vi "VBus Set from X Y Rot Angle Inputs_Cartesian.vi"(6 "Rotation":dbl, 7 "Gyro Angle":dbl, 8 "Error":errorcluster, 9 "Y":dbl, 10 "X":dbl, 11 "RobotDriveDevRef":T1={"DevStatus"={"status"=FALSE, "code"=0, "source"=""}, "Motors[]"=[], "Square Inputs"=FALSE, "Max Output"=1.0}) -> (0 "Error Out":errorcluster, 3 "RobotDriveDevRef Out":T1={"DevStatus"={"status"=FALSE, "code"=0, "source"=""}, "Motors[]"=[], "Square Inputs"=FALSE, "Max Output"=1.0})   [LabVIEW 2017, in "MechamunDrive.lvlib"]
doc: "Configures the motors for holonomic driving. Holonomic driving allows you to move the robot in any direction without first rotating or maneuvering the robot.\n\nThis VI requires the robot to have either four omni-directional wheels and four motors mounted at 45 degree angles in the four corners of a square frame or to have four mecanum wheels driven by four motors.\n\nThe control input is intended to be connected directly to the X, Y, and Z axes of a joystick. The Y axis is inverted for you.\n\nThis software is licensed. Open the labview\\readme\\WPI Robotics Library Open Source License.txt file for more information."
uses:
  MechamunDrive.lvlib
  <vilib>/Rock Robotics/WPI/RobotDrive/WPI_RobotDriveDevRef.ctl
  <vilib>/Rock Robotics/WPI/MotorControl/WPI_MotorControlDeviceRef.ctl
  <vilib>/Rock Robotics/WPI/MotorControl/WPI_MotorControlType.ctl
  <vilib>/Rock Robotics/SystemInterfaces/DIO/FPGA_DIOPWMChannel.ctl
  <vilib>/Rock Robotics/WPI/PWM/WPI_PWMDeadband.ctl
  <vilib>/Rock Robotics/SystemInterfaces/DIO/FPGA_DIOChannel.ctl
  <vilib>/Rock Robotics/SystemInterfaces/NetworkCommunication/NetComm_UsageReport_ResourceType.ctl
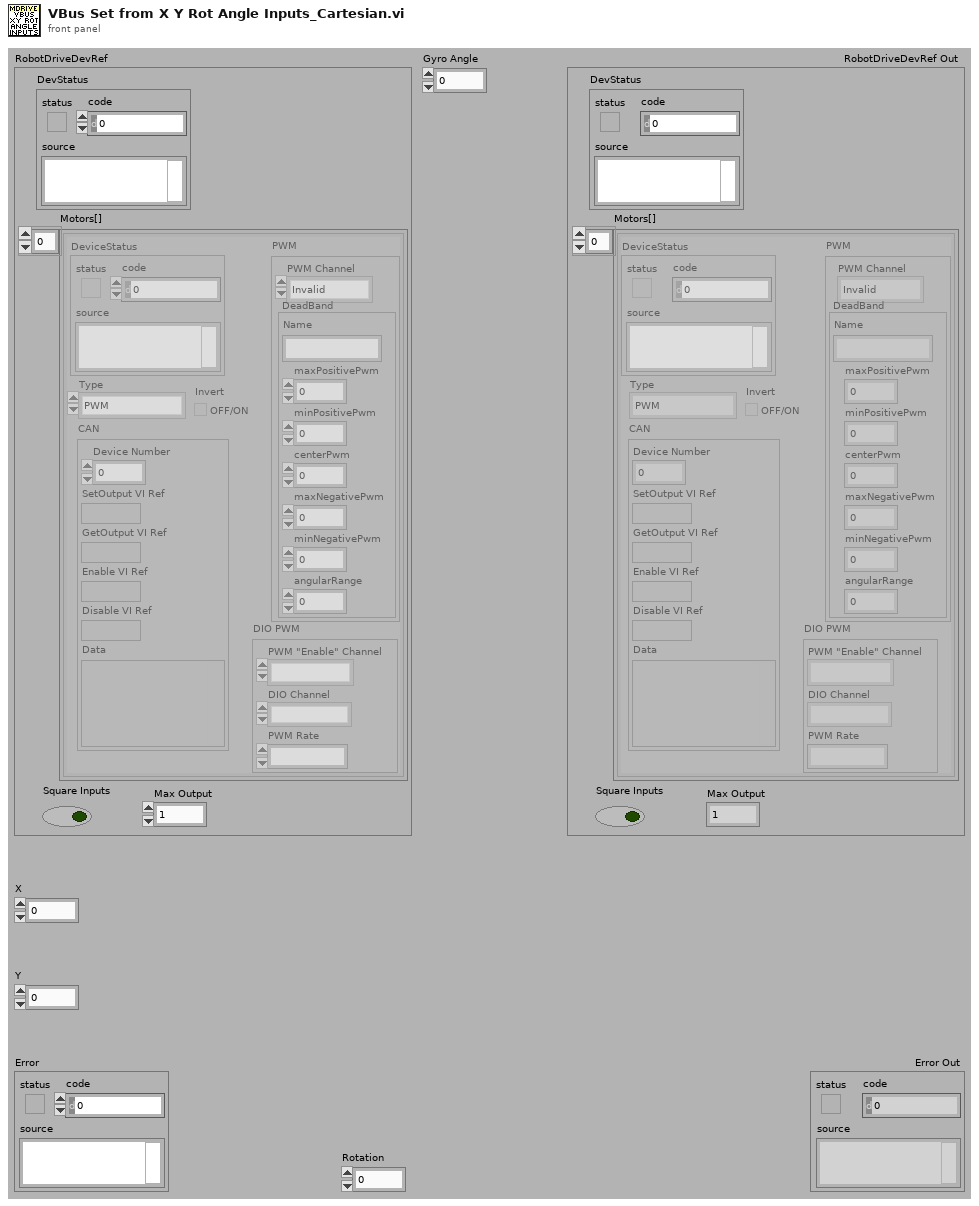
[diagram p1: front panel]
types:
  T1 = typedef "WPI_RobotDriveDevRef.ctl" = cluster{"DevStatus":errorcluster, "Motors[]":T2[], "Square Inputs":bool, "Max Output":dbl}
  T2 = typedef "WPI_MotorControlDeviceRef.ctl" = cluster{"DeviceStatus":errorcluster, "Type":T3, "PWM":cluster{"PWM Channel":T4, "DeadBand":T5}, "CAN":cluster{"Device Number":u8, "SetOutput VI Ref":variant, "GetOutput VI Ref":variant, "Enable VI Ref":variant, "Disable VI Ref":variant, "Data":variant}, "Invert":bool, "DIO PWM":cluster{"PWM \"Enable\" Channel":T4, "DIOChannel":T6, "PWM Rate":dbl}}
  T3 = typedef "WPI_MotorControlType.ctl" = enum16{"PWM", "CAN", "DIO PWM"}
  T4 = typedef "FPGA_DIOPWMChannel.ctl" = enum8{"PWM 0", "PWM 1", "PWM 2", "PWM 3", "PWM 4", "PWM 5", "PWM 6", "PWM 7", "PWM 8", "PWM 9", "PWM MXP 0", "PWM MXP 1", "PWM MXP 2", "PWM MXP 3", "PWM MXP 4", "PWM MXP 5", "PWM MXP 6", "PWM MXP 7", "PWM MXP 8", "PWM MXP 9", "Invalid"}
  T5 = typedef "WPI_PWMDeadband.ctl" = cluster{"Name":string, "maxPositivePwm":i32, "minPositivePwm":i32, "centerPwm":i32, "maxNegativePwm":i32, "minNegativePwm":i32, "angularRange":u16}
  T6 = typedef "FPGA_DIOChannel.ctl" = enum8{"DIO 0", "DIO 1", "DIO 2", "DIO 3", "DIO 4", "DIO 5", "DIO 6", "DIO 7", "DIO 8", "DIO 9", "DIO MXP 0", "DIO MXP 1", "DIO MXP 2", "DIO MXP 3", "DIO MXP 4", "DIO MXP 5", "DIO MXP 6", "DIO MXP 7", "DIO MXP 8", "DIO MXP 9", "DIO MXP 10", "DIO MXP 11", "DIO MXP 12", "DIO MXP 13", "DIO MXP 14", "DIO MXP 15", "SPI Port CS1", "SPI Port CS2", "SPI Port CS3", "SPI Port MISO", "SPI Port MOSI", "Invalid"}
  T7 = typedef "NetComm_UsageReport_ResourceType.ctl" = enum8{"Controller", "Module", "Language", "CANPlugin", "Accelerometer", "ADXL345", "AnalogChannel", "AnalogTrigger", "AnalogTriggerOutput", "CANJaguar", "Compressor", "Counter", "Dashboard", "DigitalInput", "DigitalOutput", "DriverStationCIO", "DriverStationEIO", "DriverStationLCD", "Encoder", "GearTooth", "Gyro", "I2C", "Framework", "Jaguar", "Joystick", "Kinect", "KinectStick", "PIDController", "Preferences", "PWM", "Relay", "RobotDrive", "SerialPort", "Servo", "Solenoid", "SPI", "Task", "Ultrasonic", "Victor", "Button", "Command", "AxisCamera", "PCVideoServer", "SmartDashboard", "Talon", "HiTechnicColorSensor", "HiTechnicAccel", "HiTechnicCompass", "SRF08", "AnalogOutput", "Victor SP", "Talon SRX", "CAN Talon SRX", "ADXL362 Accel", "ADXRS450 Gyro", "Rev SPARK", "Mindsensors SD540", "Digital Filter", "ADIS16448", "PDP", "PCM", "PigeonIMU", "Nidec Brushless", "CTRE CANifier", "CTRE Future 0", "CTRE Future 1", "CTRE Future 2", "CTRE Future 3", "CTRE Future 4", "CTRE Future 5", "CTRE Future 6"}
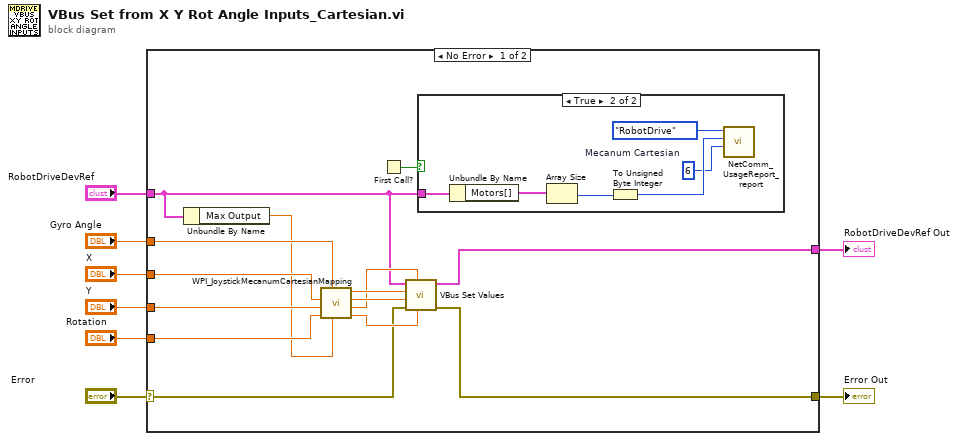
[diagram p0: block diagram]
diagram:
  n1 = case shown="No Error" "Error" {
    selector: "Error" -> [w11 w30]
    tunnel: "Y" -> [w20 _]
    tunnel: "X" -> [w19 _]
    tunnel: "RobotDriveDevRef" -> [w10 w29]
    tunnel: [w12 w29] -> w4
    tunnel: [w13 w30] -> w3
    tunnel: "Rotation" -> [w21 _]
    tunnel: "Gyro Angle" -> [w18 _]
    frame No Error {
      n2 = Unbundle By Name(w10) -> ("Max Output"=w9:dbl)
      n3 = call <vilib>:"WPI_JoystickMecanumCartesianMapping.vi"("Max Output"=w9, "Gyro Angle"=w18, "Rotation"=w21, "Y"=w20, "X"=w19) -> ("Rear Right"=w17:dbl, "Rear Left"=w14:dbl, "Front Right"=w16:dbl, "Front Left"=w15:dbl)  [unwired: 3 in]
      n4 = First Call?() -> (First Call?: T/F=w22:bool)
      n5 = call "VBus Set Values.vi"("Rear Right"=w17, "Rear Left"=w14, "error in"=w11, "Front Right"=w16, "Front Left"=w15, "RobotDriveDevRef in"=w10) -> ("error out"=w13:errorcluster, "RobotDriveDevRef out"=w12:T1)  [unwired: 4 in]
      n6 = case shown="True" w22 {
        tunnel: w10 -> [_ w23]
        frame False {
        }
        frame True {
          w26 = u8 6  # Mecanum Cartesian
          n7 = Unbundle By Name(w23) -> ("Motors[]"=w25:T2[])
          n8 = Array Size(array=w25) -> (size(s)=w24:i32)
          n9 = To Unsigned Byte Integer(number=w24) -> (unsigned 8bit integer=w27:u8)
          n10 = call <vilib>:"NetComm_UsageReport_report.vi"("Context"=w26, "Instance Number"=w27, "Resource Type"=NetComm_UsageReport_ResourceType."RobotDrive") -> ()  [unwired: 9 in]
        }
      }
    }
    frame Error {
    }
  }
  "Error Out" <- w3
  "RobotDriveDevRef Out" <- w4
